vi "VI Tree.vi"   [LabVIEW 2016, in "Agilent 2000 3000 X-Series.lvlib"]
doc: "This is the instrument driver for the Agilent 2000 3000 X-Series oscilloscope. The VI Tree displays all the user-callable VIs of the instrument driver in an organized table."
uses:
  Agilent 2000 3000 X-Series.lvlib
  Configure/Configure Measurement Edge (Delay).vi
  Action-Status/Reset Count (Mask Test).vi
  Configure/Trigger/Configure Trigger (USB).vi
  Configure/Serial Bus/Configure Serial Bus (IIC - Trigger).vi
  Configure/Reference Waveform/Configure Reference Waveform (Operation).vi
  Configure/Math/Configure Math Function (Bus).vi
  Configure/Mask Test/Configure Mask Test (Measurement).vi
  Configure/Digital Bus/Configure Bus Definition (Bits Mask).vi
  Configure/Event Search/Configure Event Search (Serial Bus - SENT).vi
  Configure/Waveform Modulation/Configure Waveform Modulation (AM).vi
  Configure/Power Analysis/Configure Power Analysis (Efficiency).vi
  Configure/Math/Configure Clock Recovery (Constant Frequency).vi
  Configure/Jitter Analysis/Configure Jitter Measurement (N-Period to Period).vi
  Data/Read Count Measurement (Event Search).vi
  Data/Read Measurement (Switching Loss Power Analysis).vi
  Data/Read Waveforms (Multiple).vi
  Data/Read Jitter Measurement (N-Period to N-Period).vi
  Configure/Configure Timebase (Basic).vi
panel:
  # "(c) 2011-2017 National Instruments.  ALL RIGHTS RESERVED."
  # "SEE DIAGRAM\nFOR VI TREE."
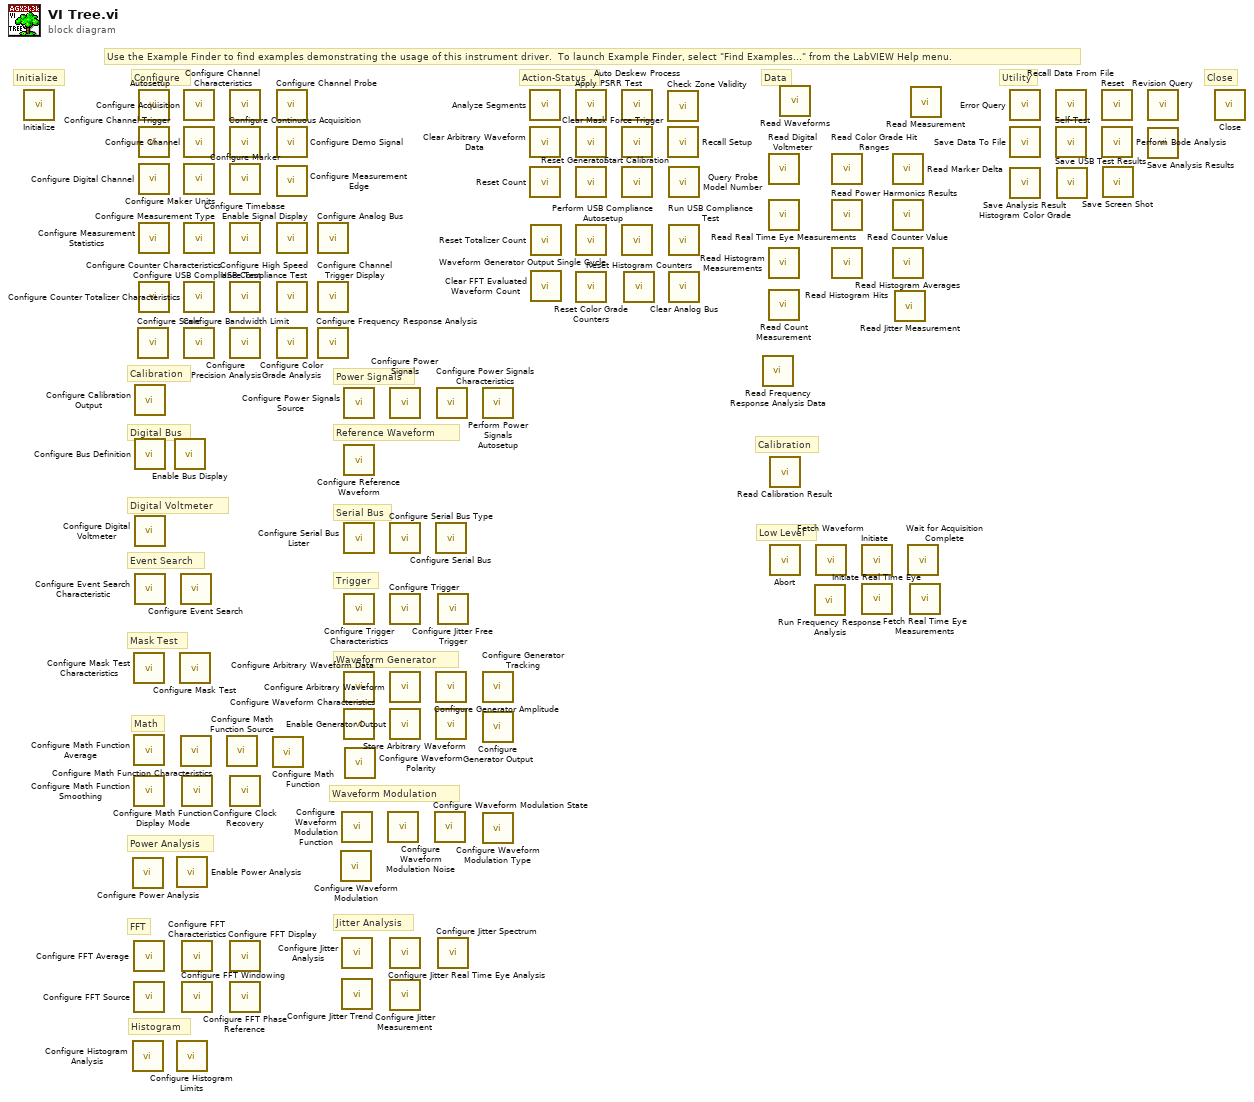
[diagram p0: block diagram]
diagram:
  # "Math"
  # "Histogram"
  # "Jitter Analysis"
  # "FFT"
  # "Waveform Modulation"
  # "Digital Voltmeter"
  # "Close"
  # "Utility"
  # "Power Analysis"
  # "Low Level"
  # "Calibration"
  # "Data"
  # "Waveform Generator"
  # "Trigger"
  # "Serial Bus"
  # "Reference Waveform"
  # "Power Signals"
  # "Mask Test"
  # "Event Search"
  # "Digital Bus"
  # "Calibration"
  # "Configure"
  # "Action-Status"
  # "Initialize"
  # "Use the Example Finder to find examples demonstrating the usage of this instrument driver.  To launch Example Finder, select \"Find Examples...\" from the LabVIEW Help menu."
  n1 = call "Initialize.vi"() -> ()  [unwired: 10 in, 2 out]
  n2 = call-poly "Configure Power Analysis.vi"() -> ()  [unwired: 10 in, 2 out]
  n3 = call "Configure Histogram Analysis.vi"() -> ()  [unwired: 10 in, 2 out]
  n4 = call "Configure Mask Test Characteristics.vi"() -> ()  [unwired: 14 in, 2 out]
  n5 = call "Configure Math Function Average.vi"() -> ()  [unwired: 10 in, 2 out]
  n6 = call "Configure Math Function Smoothing.vi"() -> ()  [unwired: 10 in, 2 out]
  n7 = call "Configure FFT Average.vi"() -> ()  [unwired: 10 in, 2 out]
  n8 = call "Configure FFT Source.vi"() -> ()  [unwired: 10 in, 2 out]
  n9 = call "Configure Calibration Output.vi"() -> ()  [unwired: 10 in, 2 out]
  n10 = call-poly "Configure Bus Definition.vi"() -> ()  [unwired: 10 in, 2 out]
  n11 = call "Configure Digital Voltmeter.vi"() -> ()  [unwired: 10 in, 2 out]
  n12 = call "Configure Event Search Characteristic.vi"() -> ()  [unwired: 10 in, 2 out]
  n13 = call "Configure Scale.vi"() -> ()  [unwired: 10 in, 2 out]
  n14 = call "Autosetup.vi"() -> ()  [unwired: 10 in, 2 out]
  n15 = call "Configure Channel Trigger.vi"() -> ()  [unwired: 10 in, 2 out]
  n16 = call "Configure Digital Channel.vi"() -> ()  [unwired: 10 in, 2 out]
  n17 = call "Configure Measurement Statistics.vi"() -> ()  [unwired: 10 in, 2 out]
  n18 = call "Configure Counter Characteristics.vi"() -> ()  [unwired: 14 in, 2 out]
  n19 = call "Enable Bus Display.vi"() -> ()  [unwired: 10 in, 2 out]
  n20 = call "Enable Power Analysis.vi"() -> ()  [unwired: 10 in, 2 out]
  n21 = call "Configure Histogram Limits.vi"() -> ()  [unwired: 10 in, 2 out]
  n22 = call-poly "Configure Mask Test.vi"() -> ()  [unwired: 14 in, 2 out]
  n23 = call-poly "Configure Event Search.vi"() -> ()  [unwired: 10 in, 2 out]
  n24 = call "Configure Math Function Characteristics.vi"() -> ()  [unwired: 14 in, 2 out]
  n25 = call "Configure Math Function Display Mode.vi"() -> ()  [unwired: 10 in, 2 out]
  n26 = call "Configure FFT Characteristics.vi"() -> ()  [unwired: 14 in, 2 out]
  n27 = call "Configure FFT Windowing.vi"() -> ()  [unwired: 10 in, 2 out]
  n28 = call "Configure Acquisition.vi"() -> ()  [unwired: 10 in, 2 out]
  n29 = call "Configure Channel.vi"() -> ()  [unwired: 14 in, 2 out]
  n30 = call "Configure Maker Units.vi"() -> ()  [unwired: 10 in, 2 out]
  n31 = call "Configure Measurement Type.vi"() -> ()  [unwired: 14 in, 2 out]
  n32 = call "Configure Counter Totalizer Characteristics.vi"() -> ()  [unwired: 14 in, 2 out]
  n33 = call "Configure Bandwidth Limit.vi"() -> ()  [unwired: 10 in, 2 out]
  n34 = call "Configure Math Function Source.vi"() -> ()  [unwired: 10 in, 2 out]
  n35 = call "Configure Channel Characteristics.vi"() -> ()  [unwired: 10 in, 2 out]
  n36 = call "Configure Continuous Acquisition.vi"() -> ()  [unwired: 10 in, 2 out]
  n37 = call "Configure Marker.vi"() -> ()  [unwired: 14 in, 2 out]
  n38 = call-poly "Configure Timebase.vi"() -> ()  [unwired: 14 in, 2 out]
  n39 = call "Configure USB Compliance Test.vi"() -> ()  [unwired: 10 in, 2 out]
  n40 = call "Configure Precision Analysis.vi"() -> ()  [unwired: 10 in, 2 out]
  n41 = call-poly "Configure Clock Recovery.vi"() -> ()  [unwired: 10 in, 2 out]
  n42 = call "Configure FFT Display.vi"() -> ()  [unwired: 10 in, 2 out]
  n43 = call "Configure FFT Phase Reference.vi"() -> ()  [unwired: 10 in, 2 out]
  n44 = call-poly "Configure Math Function.vi"() -> ()  [unwired: 10 in, 2 out]
  n45 = call "Configure Channel Probe.vi"() -> ()  [unwired: 10 in, 2 out]
  n46 = call "Configure Demo Signal.vi"() -> ()  [unwired: 10 in, 2 out]
  n47 = call-poly "Configure Measurement Edge.vi"() -> ()  [unwired: 10 in, 2 out]
  n48 = call "Enable Signal Display.vi"() -> ()  [unwired: 10 in, 2 out]
  n49 = call "Configure High Speed USB Compliance Test.vi"() -> ()  [unwired: 10 in, 2 out]
  n50 = call "Configure Color Grade Analysis .vi"() -> ()  [unwired: 10 in, 2 out]
  n51 = call "Configure Analog Bus.vi"() -> ()  [unwired: 10 in, 2 out]
  n52 = call "Configure Channel Trigger Display.vi"() -> ()  [unwired: 10 in, 2 out]
  n53 = call "Configure Frequency Response Analysis.vi"() -> ()  [unwired: 14 in, 2 out]
  n54 = call-poly "Configure Waveform Modulation.vi"() -> ()  [unwired: 10 in, 2 out]
  n55 = call "Configure Waveform Modulation Function.vi"() -> ()  [unwired: 10 in, 2 out]
  n56 = call "Configure Jitter Analysis.vi"() -> ()  [unwired: 10 in, 2 out]
  n57 = call "Configure Jitter Trend.vi"() -> ()  [unwired: 10 in, 2 out]
  n58 = call "Configure Power Signals Source.vi"() -> ()  [unwired: 10 in, 2 out]
  n59 = call-poly "Configure Reference Waveform.vi"() -> ()  [unwired: 10 in, 2 out]
  n60 = call "Configure Serial Bus Lister.vi"() -> ()  [unwired: 10 in, 2 out]
  n61 = call "Configure Trigger Characteristics.vi"() -> ()  [unwired: 14 in, 2 out]
  n62 = call "Configure Arbitrary Waveform Data.vi"() -> ()  [unwired: 10 in, 2 out]
  n63 = call "Configure Waveform Characteristics.vi"() -> ()  [unwired: 14 in, 2 out]
  n64 = call "Configure Waveform Polarity.vi"() -> ()  [unwired: 10 in, 2 out]
  n65 = call "Configure Waveform Modulation Noise.vi"() -> ()  [unwired: 10 in, 2 out]
  n66 = call "Configure Power Signals.vi"() -> ()  [unwired: 14 in, 2 out]
  n67 = call "Configure Serial Bus Type.vi"() -> ()  [unwired: 10 in, 2 out]
  n68 = call-poly "Configure Trigger.vi"() -> ()  [unwired: 10 in, 2 out]
  n69 = call "Configure Arbitrary Waveform.vi"() -> ()  [unwired: 10 in, 2 out]
  n70 = call "Enable Generator Output.vi"() -> ()  [unwired: 10 in, 2 out]
  n71 = call "Configure Jitter Real Time Eye Analysis.vi"() -> ()  [unwired: 10 in, 2 out]
  n72 = call-poly "Configure Jitter Measurement.vi"() -> ()  [unwired: 10 in, 2 out]
  n73 = call "Configure Waveform Modulation State.vi"() -> ()  [unwired: 10 in, 2 out]
  n74 = call-poly "Configure Serial Bus.vi"() -> ()  [unwired: 14 in, 2 out]
  n75 = call "Configure Generator Amplitude.vi"() -> ()  [unwired: 14 in, 2 out]
  n76 = call "Store Arbitrary Waveform.vi"() -> ()  [unwired: 10 in, 2 out]
  n77 = call "Configure Power Signals Characteristics.vi"() -> ()  [unwired: 14 in, 2 out]
  n78 = call "Configure Jitter Free Trigger.vi"() -> ()  [unwired: 10 in, 2 out]
  n79 = call "Configure Jitter Spectrum.vi"() -> ()  [unwired: 14 in, 2 out]
  n80 = call "Perform Power Signals Autosetup.vi"() -> ()  [unwired: 10 in, 2 out]
  n81 = call "Configure Generator Tracking.vi"() -> ()  [unwired: 10 in, 2 out]
  n82 = call "Configure Generator Output.vi"() -> ()  [unwired: 10 in, 2 out]
  n83 = call "Configure Waveform Modulation Type.vi"() -> ()  [unwired: 10 in, 2 out]
  n84 = call "Analyze Segments.vi"() -> ()  [unwired: 10 in, 2 out]
  n85 = call "Clear Arbitrary Waveform Data.vi"() -> ()  [unwired: 10 in, 2 out]
  n86 = call-poly "Reset Count.vi"() -> ()  [unwired: 10 in, 2 out]
  n87 = call "Reset Totalizer Count.vi"() -> ()  [unwired: 10 in, 2 out]
  n88 = call "Clear FFT Evaluated Waveform Count.vi"() -> ()  [unwired: 10 in, 2 out]
  n89 = call "Apply PSRR Test.vi"() -> ()  [unwired: 10 in, 2 out]
  n90 = call "Clear Mask.vi"() -> ()  [unwired: 10 in, 2 out]
  n91 = call "Reset Generator.vi"() -> ()  [unwired: 10 in, 2 out]
  n92 = call "Waveform Generator Output Single Cycle.vi"() -> ()  [unwired: 14 in, 2 out]
  n93 = call "Reset Color Grade Counters.vi"() -> ()  [unwired: 10 in, 2 out]
  n94 = call "Auto Deskew Process.vi"() -> ()  [unwired: 10 in, 2 out]
  n95 = call "Force Trigger.vi"() -> ()  [unwired: 10 in, 2 out]
  n96 = call "Start Calibration.vi"() -> ()  [unwired: 10 in, 2 out]
  n97 = call "Perform USB Compliance Autosetup.vi"() -> ()  [unwired: 10 in, 2 out]
  n98 = call "Reset Histogram Counters.vi"() -> ()  [unwired: 10 in, 2 out]
  n99 = call "Check Zone Validity.vi"() -> ()  [unwired: 9 in, 3 out]
  n100 = call "Recall Setup.vi"() -> ()  [unwired: 10 in, 2 out]
  n101 = call "Query Probe Model Number.vi"() -> ()  [unwired: 13 in, 3 out]
  n102 = call "Run USB Compliance Test.vi"() -> ()  [unwired: 10 in, 2 out]
  n103 = call "Clear Analog Bus.vi"() -> ()  [unwired: 10 in, 2 out]
  n104 = call "Read Frequency Response Analysis Data.vi"() -> ()  [unwired: 9 in, 3 out]
  n105 = call "Read Digital Voltmeter.vi"() -> ()  [unwired: 8 in, 4 out]
  n106 = call "Read Real Time Eye Measurements.vi"() -> ()  [unwired: 7 in, 5 out]
  n107 = call "Read Histogram Measurements.vi"() -> ()  [unwired: 9 in, 7 out]
  n108 = call-poly "Read Count Measurement.vi"() -> ()  [unwired: 9 in, 3 out]
  n109 = call "Read Calibration Result.vi"() -> ()  [unwired: 6 in, 6 out]
  n110 = call "Abort.vi"() -> ()  [unwired: 10 in, 2 out]
  n111 = call-poly "Read Waveforms.vi"() -> ()  [unwired: 9 in, 3 out]
  n112 = call "Run Frequency Response Analysis.vi"() -> ()  [unwired: 10 in, 2 out]
  n113 = call "Fetch Waveform.vi"() -> ()  [unwired: 9 in, 3 out]
  n114 = call "Read Color Grade Hit Ranges.vi"() -> ()  [unwired: 9 in, 3 out]
  n115 = call "Read Power Harmonics Results.vi"() -> ()  [unwired: 9 in, 3 out]
  n116 = call "Read Histogram Hits.vi"() -> ()  [unwired: 9 in, 7 out]
  n117 = call "Initiate.vi"() -> ()  [unwired: 10 in, 2 out]
  n118 = call "Initiate Real Time Eye.vi"() -> ()  [unwired: 10 in, 2 out]
  n119 = call "Read Marker Delta.vi"() -> ()  [unwired: 8 in, 4 out]
  n120 = call "Read Counter Value.vi"() -> ()  [unwired: 13 in, 3 out]
  n121 = call "Read Histogram Averages.vi"() -> ()  [unwired: 7 in, 5 out]
  n122 = call-poly "Read Jitter Measurement.vi"() -> ()  [unwired: 9 in, 3 out]
  n123 = call "Wait for Acquisition Complete.vi"() -> ()  [unwired: 10 in, 2 out]
  n124 = call "Fetch Real Time Eye Measurements.vi"() -> ()  [unwired: 7 in, 5 out]
  n125 = call-poly "Read Measurement.vi"() -> ()  [unwired: 13 in, 3 out]
  n126 = call "Error Query.vi"() -> ()  [unwired: 8 in, 4 out]
  n127 = call "Save Data To File.vi"() -> ()  [unwired: 14 in, 2 out]
  n128 = call "Save Analysis Result Histogram Color Grade.vi"() -> ()  [unwired: 10 in, 2 out]
  n129 = call "Recall Data From File.vi"() -> ()  [unwired: 10 in, 2 out]
  n130 = call "Self-Test.vi"() -> ()  [unwired: 8 in, 4 out]
  n131 = call "Save USB Test Results.vi"() -> ()  [unwired: 10 in, 2 out]
  n132 = call "Reset.vi"() -> ()  [unwired: 10 in, 2 out]
  n133 = call "Perform Bode Analysis.vi"() -> ()  [unwired: 10 in, 2 out]
  n134 = call "Save Screen Shot.vi"() -> ()  [unwired: 10 in, 2 out]
  n135 = call "Revision Query.vi"() -> ()  [unwired: 8 in, 4 out]
  n136 = call "Save Analysis Results.vi"() -> ()  [unwired: 14 in, 2 out]
  n137 = call "Close.vi"() -> ()  [unwired: 11 in, 1 out]
